vi "diff-freq.vi"() -> ()   [LabVIEW 2019]
uses:
  <vilib>/DAQmx/create/channels.llb/DAQmx Create Channel (CO-Pulse Generation-Ticks).vi
  <vilib>/DAQmx/configure/timing.llb/DAQmx Timing (Implicit).vi
  <resource>/objmgr/daqmx.rc
panel:
  in  "stop":bool
  out "CO.CtrTimebaseRate":dbl
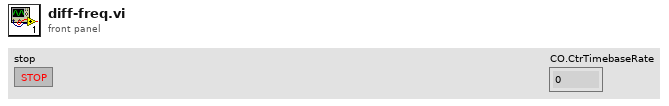
[diagram p1: front panel]
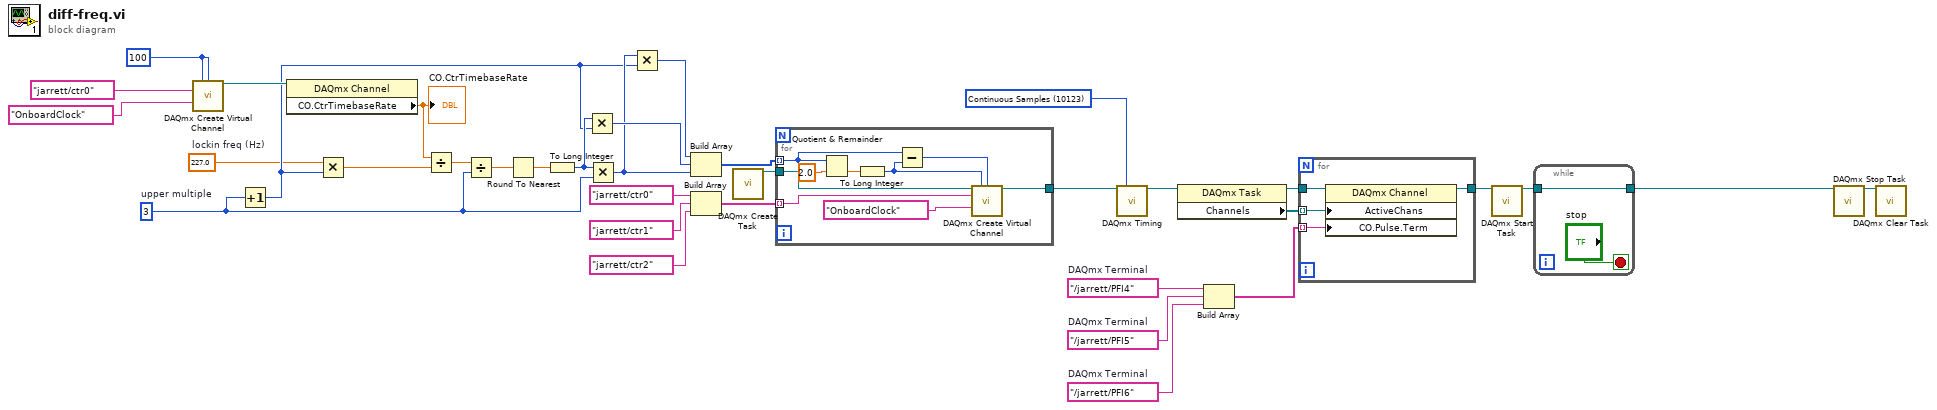
[diagram p0: block diagram]
diagram:
  w3 = 10123 items=["Finite Samples"=10178, "Continuous Samples"=10123, "Hardware Timed Single Point"=12522] ("sample mode")
  w7 = tag "/jarrett/PFI6"  # DAQmx Terminal
  w8 = tag "/jarrett/PFI5"  # DAQmx Terminal
  w9 = tag "/jarrett/PFI4"  # DAQmx Terminal
  w29 = 3  # upper multiple
  w33 = u32 100 ("low ticks")
  w17 = 227.0  # lockin freq (Hz)
  n1 = call-poly <vilib>:"DAQmx Create Virtual Channel.vi"("high ticks"=w33, "low ticks"=w33, "counter"=tag "jarrett/ctr0", "source of ticks"=tag "OnboardClock") -> ("task out"=w32:refnum<k21>)  [unwired: 10 in, 1 out]
  n2 = Increment(x=w29) -> (x+1=w18:i32)
  n3 = property class="DAQmx Channel"(reference=w32) -> ("CO.CtrTimebaseRate"=w31:dbl)  [unwired: 1 in, 2 out]
  "CO.CtrTimebaseRate" <- w31
  n4 = Multiply(x=w17, y=w18) -> (x*y=w16:dbl)
  n5 = Divide(x=w31, y=w16) -> (x/y=w30:dbl)
  n6 = Divide(x=w30, y=w29) -> (x/y=w2:dbl)
  n7 = Round To Nearest(number=w2) -> (nearest integer value=w1:dbl)
  n8 = To Long Integer(number=w1) -> (32bit integer=w28:i32)
  n9 = Multiply(x=w28, y=w18) -> (x*y=w26:i32)
  n10 = Multiply(x=w28, y=w29) -> (x*y=w25:i32)
  n11 = Multiply(x=w25, y=w18) -> (x*y=w27:i32)
  n12 = Build Array(w27, w26, w25) -> (w21:i32[])
  n13 = Build Array(tag "jarrett/ctr0" ("counter"), tag "jarrett/ctr1" ("counter"), tag "jarrett/ctr2" ("counter")) -> (w20:tag[])
  n14 = call <vilib>:"DAQmx Create Task.vi"() -> ("task out"=w19:refnum<k21>)  [unwired: 14 in, 1 out]
  n15 = for {
    tunnel: w21 -> [w42] mode=indexing
    tunnel: w20 -> [w39] mode=indexing
    tunnel: w19 -> [w38]
    tunnel: [w36] -> w5
    n16 = Quotient & Remainder(x=w42, y=2.0) -> (floor(x/y)=w43:dbl)  [unwired: 1 out]
    n17 = To Long Integer(number=w43) -> (32bit integer=w41:i32)
    n18 = Subtract(x=w42, y=w41) -> (x-y=w40:i32)
    n19 = call-poly <vilib>:"DAQmx Create Virtual Channel.vi"("task in"=w38, "high ticks"=w41, "low ticks"=w40, "counter"=w39, "source of ticks"=tag "OnboardClock") -> ("task out"=w36:refnum<k21>)  [unwired: 9 in, 1 out]
  }
  n20 = call-poly <vilib>:"DAQmx Timing.vi"("task/channels in"=w5, "sample mode"=w3) -> ("task out"=w4:refnum<k21>)  [unwired: 12 in, 1 out]
  n21 = property class="DAQmx Task"(reference=w4) -> (reference out=w12:refnum<k21>, "Channels"=w13:refnum<k21>[])  [unwired: 1 in, 1 out]
  n22 = Build Array(w9, w8, w7) -> (w6:tag[])
  n23 = for {
    tunnel: w13 -> [w47] mode=indexing
    tunnel: w12 -> [w48]
    tunnel: [w46] -> w10
    tunnel: w6 -> [w45] mode=indexing
    n24 = property class="DAQmx Channel"(reference=w48, "ActiveChans"=w47, "CO.Pulse.Term"=w45) -> (reference out=w46:refnum<k21>)  [unwired: 1 in, 1 out]
  }
  n25 = call <vilib>:"DAQmx Start Task.vi"("task/channels in"=w10) -> ("task out"=w11:refnum<k21>)  [unwired: 13 in, 1 out]
  n26 = while {
    tunnel: [w49] -> w15
    tunnel: w11 -> [w49]
    stop <- "stop" stop-if-true
  }
  n27 = call <vilib>:"DAQmx Stop Task.vi"("task/channels in"=w15) -> ("task out"=w14:refnum<k21>)  [unwired: 13 in, 1 out]
  n28 = call <vilib>:"DAQmx Clear Task.vi"("task in"=w14) -> ()  [unwired: 14 in, 1 out]
